vi "Initialization VI.vi"(8 "error in (no error)":errorcluster, 10 "Custom XML":string, 11 "Device Item Ref in":T1 format="%.0x") -> (0 "error out":errorcluster, 3 "Device Item Ref out":T1 format="%.0x")   [LabVIEW 2015, in "Fuel Injection Addon System Explorer.lvlib"]
uses:
  Fuel Injection Addon System Explorer.lvlib
  <vilib>/NI Veristand/Custom Device API/Custom Device Item Ref.ctl
  <vilib>/NI Veristand/Custom Device API/Custom Device Channel.ctl
  <vilib>/NI Veristand/Custom Device API/Custom Device Channel Type.ctl
  Shared/Constants.vi
  <vilib>/NI VeriStand/Custom Device API/Custom Device API.lvlib
  Shared/Fuel Injection Addon Shared.lvlib
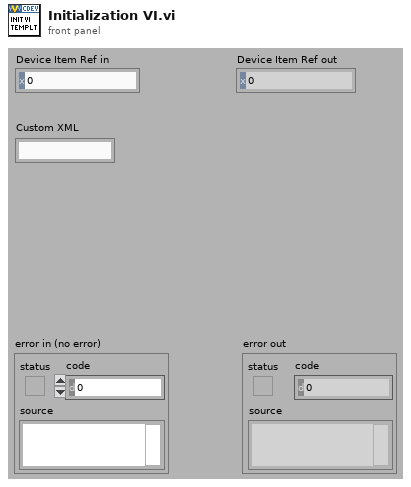
[diagram p1: front panel]
types:
  T1 = typedef "Custom Device API.lvlib/Custom Device Item Ref.ctl" = u64
  T2 = typedef "Custom Device API.lvlib/Custom Device Channel.ctl" = cluster{"Type":T3, "Units":string, "Default Value":dbl, "Faultable":bool, "Scalable":bool}
  T3 = typedef "Custom Device API.lvlib/Custom Device Channel Type.ctl" = enum16{"Input", "Output"}
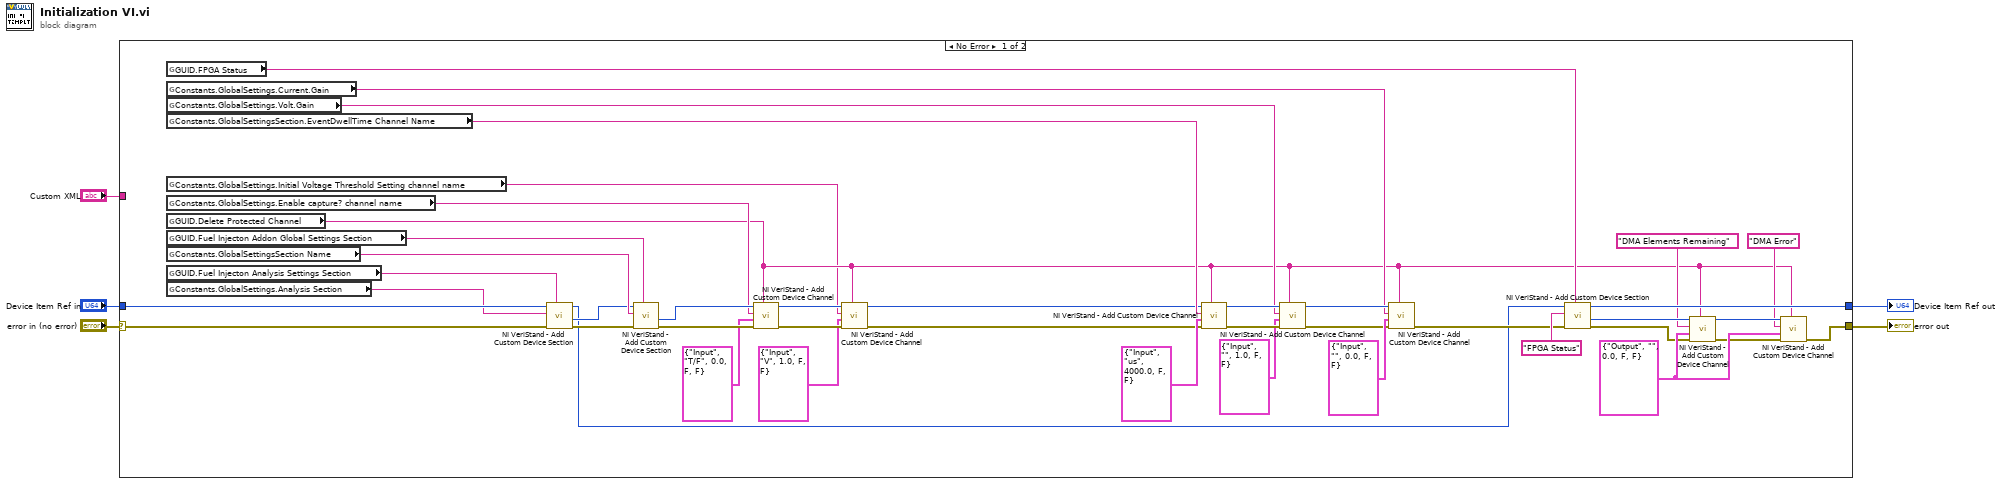
[diagram p0: block diagram]
diagram:
  n1 = case shown="No Error" "error in (no error)" {
    selector: "error in (no error)" -> [w19 w49]
    tunnel: [w29 w49] -> w5
    tunnel: [w35 w48] -> w3
    tunnel: "Device Item Ref in" -> [w17 w48]
    tunnel: "Custom XML" -> [_ _]
    frame No Error {
      w32 = T2 {"Type"=enum."Output", "Units"="", "Default Value"=0.0, "Faultable"=FALSE, "Scalable"=FALSE} ("Channel")
      n2 = global read "Constants.vi" "GUID.FPGA Status"() -> (w34:string)
      n3 = global read "Constants.vi" "Constants.GlobalSettings.Current.Gain"() -> (w21:string)
      n4 = global read "Constants.vi" "Constants.GlobalSettings.Volt.Gain"() -> (w22:string)
      n5 = global read "Constants.vi" "Constants.GlobalSettingsSection.EventDwellTime Channel Name"() -> (w23:string)
      n6 = global read "Constants.vi" "Constants.GlobalSettings.Initial Voltage Threshold Setting channel name"() -> (w8:string)
      n7 = global read "Constants.vi" "Constants.GlobalSettings.Enable capture? channel name"() -> (w24:string)
      n8 = global read "Constants.vi" "GUID.Delete Protected Channel"() -> (w9:string)
      n9 = global read "Constants.vi" "GUID.Fuel Injecton Addon Global Settings Section"() -> (w47:string)
      n10 = global read "Constants.vi" "Constants.GlobalSettingsSection Name"() -> (w44:string)
      n11 = global read "Constants.vi" "GUID.Fuel Injecton Analysis Settings Section"() -> (w15:string)
      n12 = global read "Constants.vi" "Constants.GlobalSettings.Analysis Section"() -> (w16:string)
      n13 = call <vilib>:"NI VeriStand - Add Custom Device Section.vi"("GUID (Default Section)"=w15, "error in (no error)"=w19, "Section Name"=w16, "Parent Ref in"=w17) -> ("error out"=w18:errorcluster, "Section Ptr"=w14:T1, "Parent Ref out"=w13:T1)  [unwired: 4 in, 1 out]
      n14 = call <vilib>:"NI VeriStand - Add Custom Device Section.vi"("GUID (Default Section)"=w47, "error in (no error)"=w18, "Section Name"=w44, "Parent Ref in"=w14) -> ("error out"=w46:errorcluster, "Section Ptr"=w45:T1)  [unwired: 4 in, 2 out]
      n15 = call <vilib>:"NI VeriStand - Add Custom Device Channel.vi"("GUID (Default Channel)"=w9, "error in (no error)"=w46, "Channel"=T2 {"Type"=enum."Input", "Units"="T/F", "Default Value"=0.0, "Faultable"=FALSE, "Scalable"=FALSE}, "Channel Name"=w24, "Parent Ref in"=w45) -> ("error out"=w12:errorcluster, "Parent Ref out"=w11:T1)  [unwired: 3 in, 2 out]
      n16 = call <vilib>:"NI VeriStand - Add Custom Device Channel.vi"("GUID (Default Channel)"=w9, "error in (no error)"=w12, "Channel"=T2 {"Type"=enum."Input", "Units"="V", "Default Value"=1.0, "Faultable"=FALSE, "Scalable"=FALSE}, "Channel Name"=w8, "Parent Ref in"=w11) -> ("error out"=w7:errorcluster, "Parent Ref out"=w6:T1)  [unwired: 3 in, 2 out]
      n17 = call <vilib>:"NI VeriStand - Add Custom Device Channel.vi"("GUID (Default Channel)"=w9, "error in (no error)"=w7, "Channel"=T2 {"Type"=enum."Input", "Units"="us", "Default Value"=4000.0, "Faultable"=FALSE, "Scalable"=FALSE}, "Channel Name"=w23, "Parent Ref in"=w6) -> ("error out"=w40:errorcluster, "Parent Ref out"=w41:T1)  [unwired: 3 in, 2 out]
      n18 = call <vilib>:"NI VeriStand - Add Custom Device Channel.vi"("GUID (Default Channel)"=w9, "error in (no error)"=w40, "Channel"=T2 {"Type"=enum."Input", "Units"="", "Default Value"=1.0, "Faultable"=FALSE, "Scalable"=FALSE}, "Channel Name"=w22, "Parent Ref in"=w41) -> ("error out"=w36:errorcluster, "Parent Ref out"=w37:T1)  [unwired: 3 in, 2 out]
      n19 = call <vilib>:"NI VeriStand - Add Custom Device Channel.vi"("GUID (Default Channel)"=w9, "error in (no error)"=w36, "Channel"=T2 {"Type"=enum."Input", "Units"="", "Default Value"=0.0, "Faultable"=FALSE, "Scalable"=FALSE}, "Channel Name"=w21, "Parent Ref in"=w37) -> ("error out"=w20:errorcluster)  [unwired: 3 in, 3 out]
      n20 = call <vilib>:"NI VeriStand - Add Custom Device Section.vi"("GUID (Default Section)"=w34, "error in (no error)"=w20, "Section Name"="FPGA Status", "Parent Ref in"=w13) -> ("error out"=w28:errorcluster, "Section Ptr"=w33:T1, "Parent Ref out"=w35:T1)  [unwired: 4 in, 1 out]
      n21 = call <vilib>:"NI VeriStand - Add Custom Device Channel.vi"("GUID (Default Channel)"=w9, "error in (no error)"=w28, "Channel"=w32, "Channel Name"="DMA Elements Remaining", "Parent Ref in"=w33) -> ("error out"=w31:errorcluster, "Parent Ref out"=w30:T1)  [unwired: 3 in, 2 out]
      n22 = call <vilib>:"NI VeriStand - Add Custom Device Channel.vi"("GUID (Default Channel)"=w9, "error in (no error)"=w31, "Channel"=w32, "Channel Name"="DMA Error", "Parent Ref in"=w30) -> ("error out"=w29:errorcluster)  [unwired: 3 in, 3 out]
    }
    frame Error {
    }
  }
  "error out" <- w5
  "Device Item Ref out" <- w3
